vi "SFCT Motor Control.vi"(9 "Start":bool, 10 "VISA resource":refnum<visa-resource-name>, 11 "To Position":u16(ring) items=["Staging", "Press", "Cooling", "Auto Home", "Home"]) -> (0 "Y position":dbl, 1 "X Position":dbl)   [LabVIEW 2020]
uses:
  <vilib>/LabVIEW Interface for Arduino/LabVIEW Interface for Arduino.lvlib
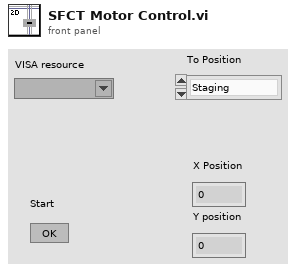
[diagram p1: front panel]
types:
  T1 = typedef "LabVIEW Interface for Arduino.lvlib/Arduino Resource.ctl" = cluster{"VISA resource":refnum<visa-resource-name>, "Board Type":T2, "Connection Type":enum8{"USB / Serial"}, "Bytes Per Packet (15)":u8}
  T2 = typedef "LabVIEW Interface for Arduino.lvlib/Board Type.ctl" = enum16{"Uno", "Dimuelanove w/Atmega 328", "Mega 2560"}
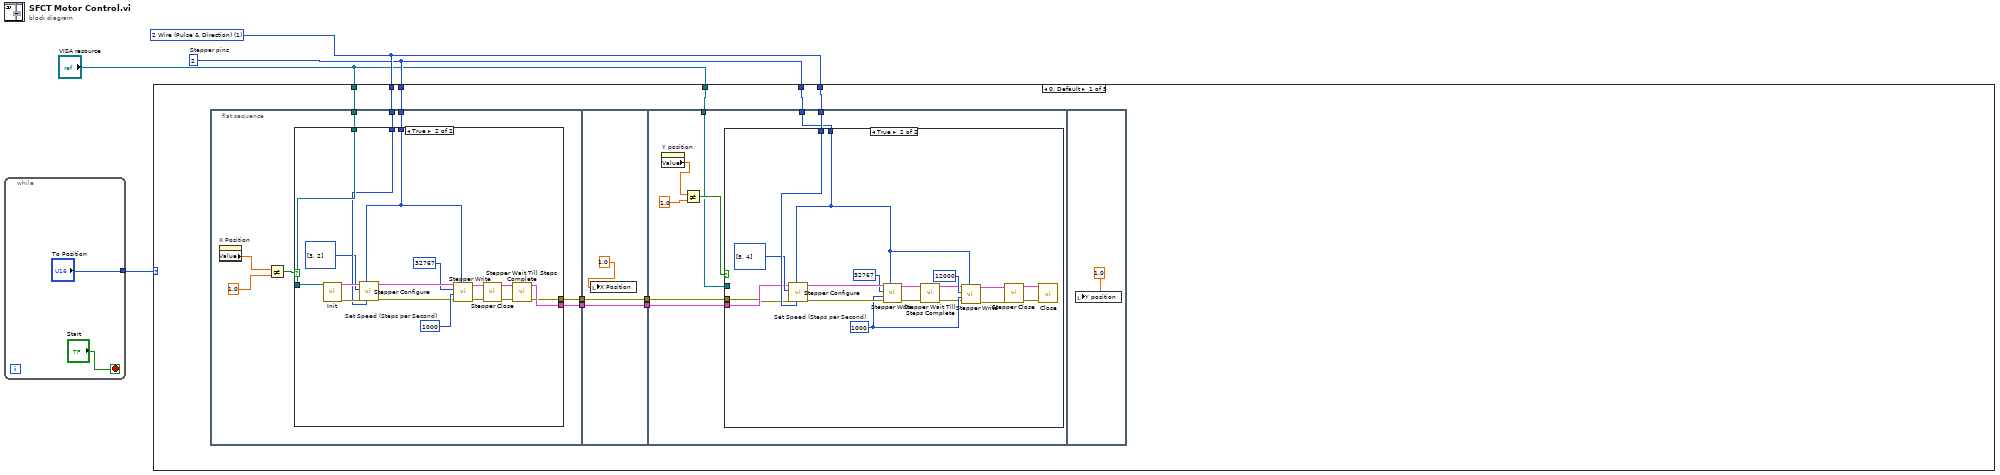
[diagram p0: block diagram]
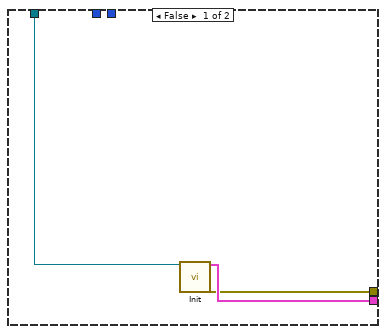
[diagram p2: hidden frame]
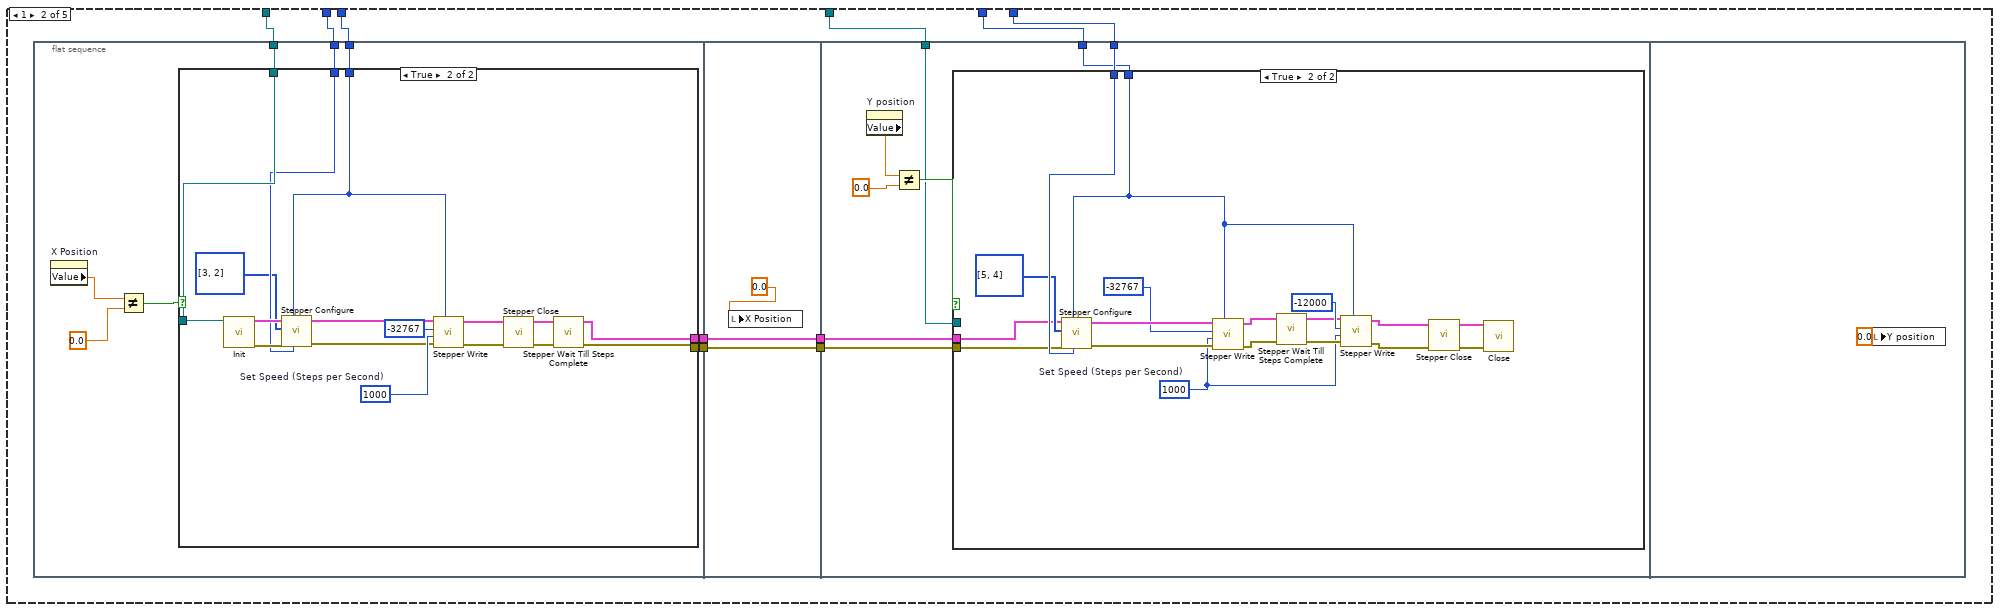
[diagram p4: hidden frame]
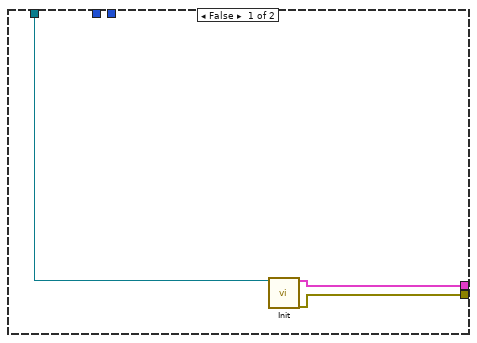
[diagram p5: hidden frame]
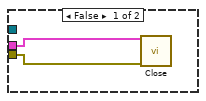
[diagram p6: hidden frame]
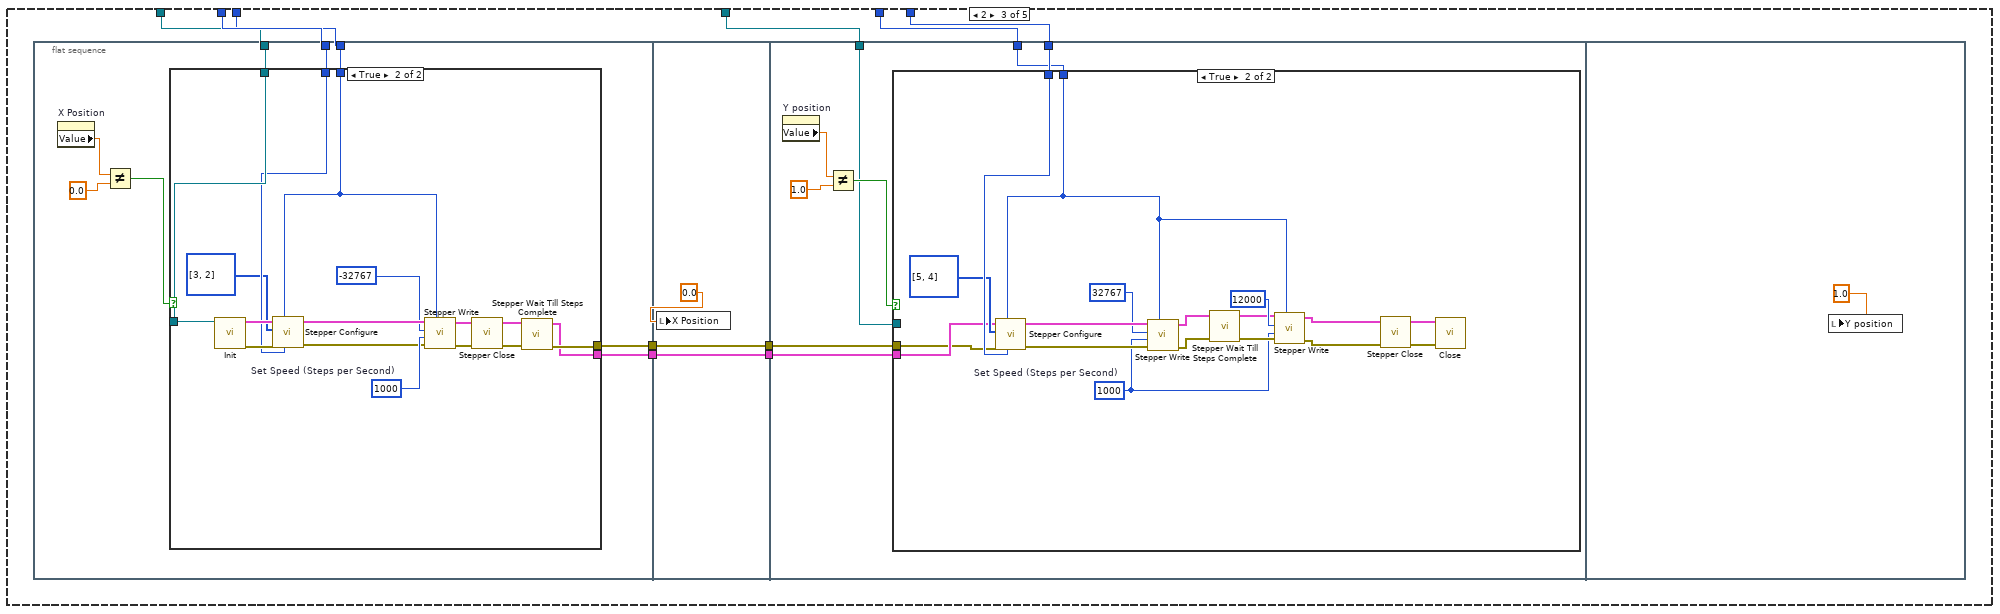
[diagram p7: hidden frame]
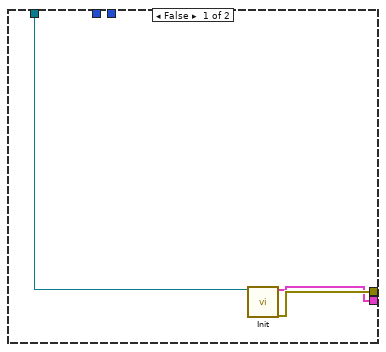
[diagram p8: hidden frame]
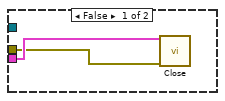
[diagram p9: hidden frame]
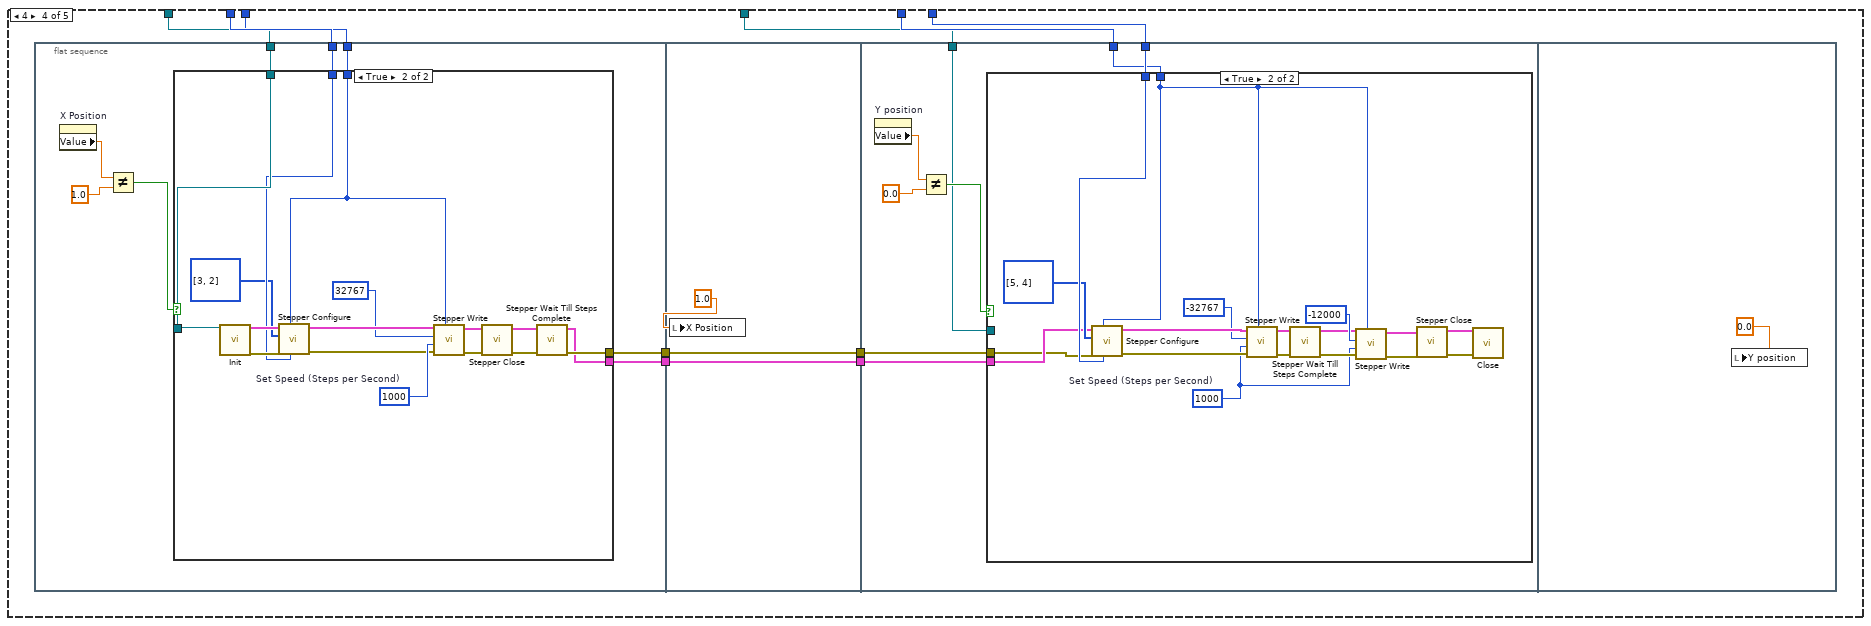
[diagram p10: hidden frame]
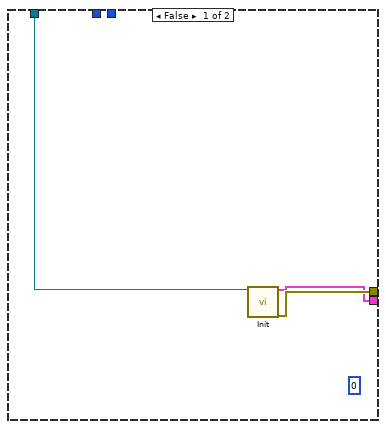
[diagram p11: hidden frame]
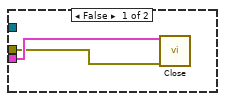
[diagram p12: hidden frame]
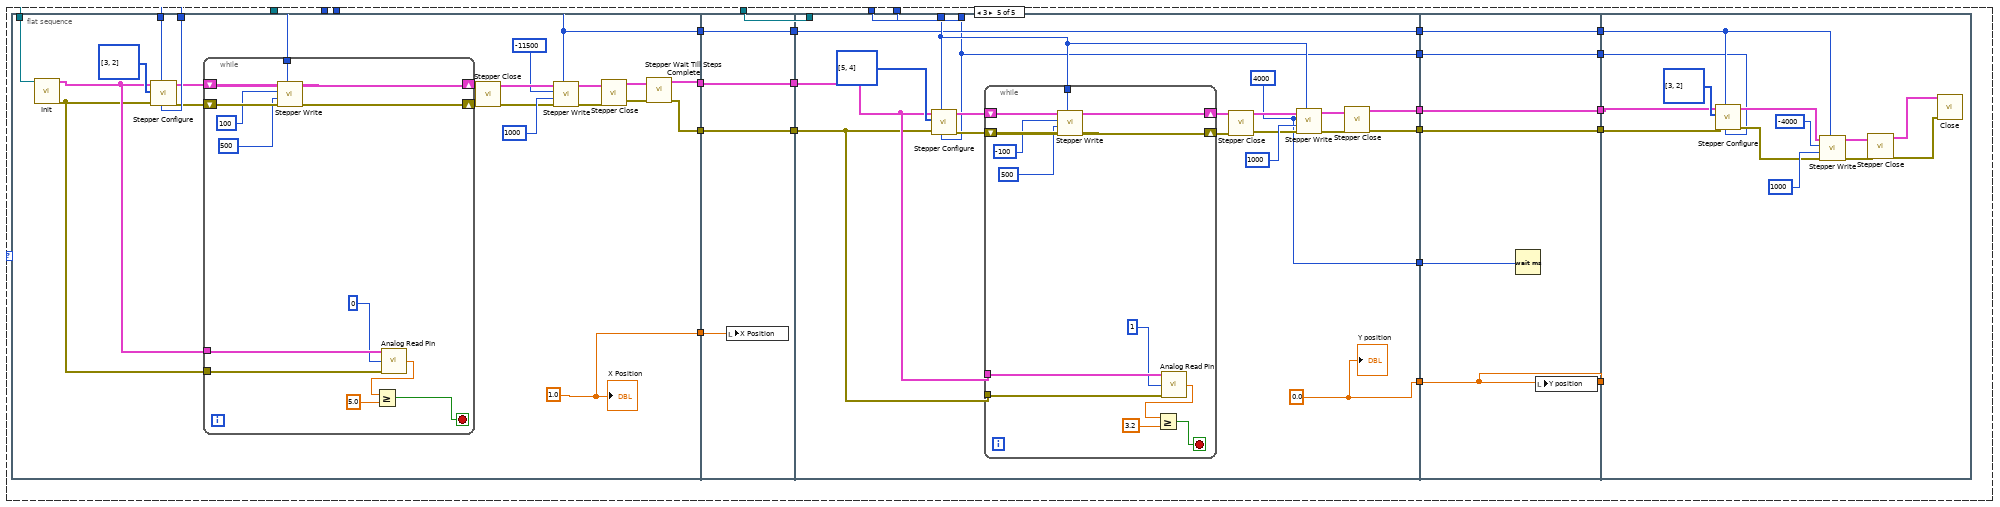
[diagram p13: hidden frame]
diagram:
  w2 = 2  # Stepper pins
  w3 = u8 1 items=["2 Wire (Pulse & Direction)"=1, "2 Wire"=2, "4 Wire"=4, "EasyDriver"=6, "AF Motor Shield (Stepper 1 & 2 Only)"=5] ("Control Method")
  n1 = while {
    tunnel: ["To Position"] -> w4
    stop <- "Start" stop-if-true
  }
  n2 = case shown="0, Default" w4 {
    tunnel: "VISA resource" -> [w11 w78 w147 w216 w301]
    tunnel: w3 -> [w13 w80 w149 w218 w300]
    tunnel: w2 -> [w12 w79 w148 w217 w299]
    tunnel: w3 -> [w16 w83 w152 w221 _]
    tunnel: w2 -> [w15 w82 w151 w220 _]
    tunnel: "VISA resource" -> [w14 w81 w150 w219 _]
    frame 0, Default {
      n3 = flat-sequence {
        tunnel: w16 -> [w23]
        tunnel: w15 -> [w22]
        tunnel: w14 -> [w19]
        tunnel: [w21] -> w9
        tunnel: [w20] -> w7
        tunnel: [w46] -> w10
        tunnel: w9 -> [w46]
        tunnel: [w45] -> w8
        tunnel: w7 -> [w45]
        tunnel: w13 -> [w53]
        tunnel: w12 -> [w52]
        tunnel: w11 -> [w51]
        tunnel: w10 -> [w50]
        tunnel: w8 -> [w49]
        frame #0 {
          n4 = property on="X Position" class="DigNum (strict)"() -> ("Value"=w17:dbl)  [unwired: 2 in, 2 out]
          n5 = Not Equal?(x=w17, y=1.0) -> (x != y?=w24:bool)
          n6 = case shown="True" w24 {
            tunnel: w23 -> [_ w40]
            tunnel: w22 -> [_ w36]
            tunnel: w19 -> [_ w33]
            tunnel: [w27 w31] -> w21
            tunnel: [w26 w30] -> w20
            tunnel: w19 -> [w25 _]
            frame False {
              n7 = call <vilib>:"Init.vi"("VISA resource"=w25) -> ("Arduino Resource"=w27:T1, "error out"=w26:errorcluster)  [unwired: 17 in]
            }
            frame True {
              w41 = i16 1000  # Set Speed (Steps per Second)
              n8 = call <vilib>:"Init.vi"("VISA resource"=w33) -> ("Arduino Resource"=w43:T1, "error out"=w42:errorcluster)  [unwired: 17 in]
              n9 = call <vilib>:"Stepper Configure.vi"("Control Method"=w40, "Stepper #"=w36, "error in"=w42, "Stepper Pins"=u8[] [3, 2], "Arduino Resource"=w43) -> ("error out"=w37:errorcluster, "Arduino Resource Out"=w38:T1)  [unwired: 5 in]
              n10 = call <vilib>:"Stepper Write.vi"("Stepper #"=w36, "error in"=w37, "Set Speed (Steps per Second)"=w41, "# of Steps to Move"=i16 32767, "Arduino Resource"=w38) -> ("error out"=w35:errorcluster, "Arduino Resource Out"=w34:T1)  [unwired: 5 in]
              n11 = call <vilib>:"Stepper Close.vi"("error in"=w35, "Arduino Resource"=w34) -> ("error out"=w29:errorcluster, "Arduino Resource Out"=w28:T1)  [unwired: 8 in]
              n12 = call <vilib>:"Stepper Wait Till Steps Complete.vi"("error in"=w29, "Arduino Resource In"=w28) -> ("error out"=w30:errorcluster, "Arduino Resource Out"=w31:T1)  [unwired: 8 in]
            }
          }
        }
        frame #1 {
          n13 = local write "X Position"(1.0 ("X Position")) -> ()
        }
        frame #2 {
          n14 = property on="Y position" class="DigNum (strict)"() -> ("Value"=w47:dbl)  [unwired: 2 in, 2 out]
          n15 = Not Equal?(x=w47, y=1.0) -> (x != y?=w54:bool)
          n16 = case shown="True" w54 {
            tunnel: w53 -> [_ w72]
            tunnel: w52 -> [_ w61]
            tunnel: w51 -> [_ _]
            tunnel: w50 -> [_ w66]
            tunnel: w49 -> [_ w65]
            frame False {
            }
            frame True {
              w60 = i16 1000  # Set Speed (Steps per Second)
              n17 = call <vilib>:"Stepper Configure.vi"("Control Method"=w72, "Stepper #"=w61, "error in"=w65, "Stepper Pins"=u8[] [5, 4], "Arduino Resource"=w66) -> ("error out"=w69:errorcluster, "Arduino Resource Out"=w70:T1)  [unwired: 5 in]
              n18 = call <vilib>:"Stepper Write.vi"("Stepper #"=w61, "error in"=w69, "Set Speed (Steps per Second)"=w60, "# of Steps to Move"=i16 32767, "Arduino Resource"=w70) -> ("error out"=w58:errorcluster, "Arduino Resource Out"=w57:T1)  [unwired: 5 in]
              n19 = call <vilib>:"Stepper Wait Till Steps Complete.vi"("error in"=w58, "Arduino Resource In"=w57) -> ("error out"=w55:errorcluster, "Arduino Resource Out"=w56:T1)  [unwired: 8 in]
              n20 = call <vilib>:"Stepper Write.vi"("Stepper #"=w61, "error in"=w55, "Set Speed (Steps per Second)"=w60, "# of Steps to Move"=i16 12000, "Arduino Resource"=w56) -> ("error out"=w63:errorcluster, "Arduino Resource Out"=w62:T1)  [unwired: 5 in]
              n21 = call <vilib>:"Stepper Close.vi"("error in"=w63, "Arduino Resource"=w62) -> ("error out"=w67:errorcluster, "Arduino Resource Out"=w68:T1)  [unwired: 8 in]
              n22 = call <vilib>:"Close.vi"("Arduino Resource"=w68, "error in"=w67) -> ()  [unwired: 13 in, 1 out]
            }
          }
        }
        frame #3 {
          n23 = local write "Y position"(1.0 ("Y position")) -> ()
        }
      }
    }
    frame 1 {
      n24 = flat-sequence {
        tunnel: w83 -> [w90]
        tunnel: w82 -> [w89]
        tunnel: w81 -> [w86]
        tunnel: [w88] -> w76
        tunnel: [w87] -> w74
        tunnel: [w113] -> w77
        tunnel: w76 -> [w113]
        tunnel: [w112] -> w75
        tunnel: w74 -> [w112]
        tunnel: w80 -> [w120]
        tunnel: w79 -> [w119]
        tunnel: w78 -> [w118]
        tunnel: w77 -> [w117]
        tunnel: w75 -> [w116]
        frame #0 {
          n25 = property on="X Position" class="DigNum (strict)"() -> ("Value"=w84:dbl)  [unwired: 2 in, 2 out]
          n26 = Not Equal?(x=w84, y=0.0) -> (x != y?=w91:bool)
          n27 = case shown="True" w91 {
            tunnel: w90 -> [_ w107]
            tunnel: w89 -> [_ w103]
            tunnel: w86 -> [_ w100]
            tunnel: [w92 w95] -> w88
            tunnel: [w93 w96] -> w87
            tunnel: w86 -> [w94 _]
            frame False {
              n28 = call <vilib>:"Init.vi"("VISA resource"=w94) -> ("Arduino Resource"=w93:T1, "error out"=w92:errorcluster)  [unwired: 17 in]
            }
            frame True {
              w108 = i16 1000  # Set Speed (Steps per Second)
              n29 = call <vilib>:"Init.vi"("VISA resource"=w100) -> ("Arduino Resource"=w110:T1, "error out"=w109:errorcluster)  [unwired: 17 in]
              n30 = call <vilib>:"Stepper Configure.vi"("Control Method"=w107, "Stepper #"=w103, "error in"=w109, "Stepper Pins"=u8[] [3, 2], "Arduino Resource"=w110) -> ("error out"=w104:errorcluster, "Arduino Resource Out"=w105:T1)  [unwired: 5 in]
              n31 = call <vilib>:"Stepper Write.vi"("Stepper #"=w103, "error in"=w104, "Set Speed (Steps per Second)"=w108, "# of Steps to Move"=i16 -32767, "Arduino Resource"=w105) -> ("error out"=w102:errorcluster, "Arduino Resource Out"=w101:T1)  [unwired: 5 in]
              n32 = call <vilib>:"Stepper Close.vi"("error in"=w102, "Arduino Resource"=w101) -> ("error out"=w97:errorcluster, "Arduino Resource Out"=w98:T1)  [unwired: 8 in]
              n33 = call <vilib>:"Stepper Wait Till Steps Complete.vi"("error in"=w97, "Arduino Resource In"=w98) -> ("error out"=w95:errorcluster, "Arduino Resource Out"=w96:T1)  [unwired: 8 in]
            }
          }
        }
        frame #1 {
          n34 = local write "X Position"(0.0 ("X Position")) -> ()
        }
        frame #2 {
          n35 = property on="Y position" class="DigNum (strict)"() -> ("Value"=w114:dbl)  [unwired: 2 in, 2 out]
          n36 = Not Equal?(x=w114, y=0.0) -> (x != y?=w121:bool)
          n37 = case shown="True" w121 {
            tunnel: w120 -> [_ w141]
            tunnel: w119 -> [_ w125]
            tunnel: w118 -> [_ _]
            tunnel: w117 -> [w122 w135]
            tunnel: w116 -> [w123 w134]
            frame False {
              n38 = call <vilib>:"Close.vi"("Arduino Resource"=w123, "error in"=w122) -> ()  [unwired: 13 in, 1 out]
            }
            frame True {
              w124 = i16 1000  # Set Speed (Steps per Second)
              n39 = call <vilib>:"Stepper Configure.vi"("Control Method"=w141, "Stepper #"=w125, "error in"=w135, "Stepper Pins"=u8[] [5, 4], "Arduino Resource"=w134) -> ("error out"=w138:errorcluster, "Arduino Resource Out"=w139:T1)  [unwired: 5 in]
              n40 = call <vilib>:"Stepper Write.vi"("Stepper #"=w125, "error in"=w138, "Set Speed (Steps per Second)"=w124, "# of Steps to Move"=i16 -32767, "Arduino Resource"=w139) -> ("error out"=w128:errorcluster, "Arduino Resource Out"=w129:T1)  [unwired: 5 in]
              n41 = call <vilib>:"Stepper Wait Till Steps Complete.vi"("error in"=w128, "Arduino Resource In"=w129) -> ("error out"=w130:errorcluster, "Arduino Resource Out"=w131:T1)  [unwired: 8 in]
              n42 = call <vilib>:"Stepper Write.vi"("Stepper #"=w125, "error in"=w130, "Set Speed (Steps per Second)"=w124, "# of Steps to Move"=i16 -12000, "Arduino Resource"=w131) -> ("error out"=w127:errorcluster, "Arduino Resource Out"=w126:T1)  [unwired: 5 in]
              n43 = call <vilib>:"Stepper Close.vi"("error in"=w127, "Arduino Resource"=w126) -> ("error out"=w136:errorcluster, "Arduino Resource Out"=w137:T1)  [unwired: 8 in]
              n44 = call <vilib>:"Close.vi"("Arduino Resource"=w137, "error in"=w136) -> ()  [unwired: 13 in, 1 out]
            }
          }
        }
        frame #3 {
          n45 = local write "Y position"(0.0 ("Y position")) -> ()
        }
      }
    }
    frame 2 {
      n46 = flat-sequence {
        tunnel: w152 -> [w159]
        tunnel: w151 -> [w158]
        tunnel: w150 -> [w155]
        tunnel: [w157] -> w145
        tunnel: [w156] -> w144
        tunnel: [w182] -> w146
        tunnel: w145 -> [w182]
        tunnel: w144 -> [w181]
        tunnel: [w181] -> w143
        tunnel: w149 -> [w189]
        tunnel: w148 -> [w188]
        tunnel: w147 -> [w187]
        tunnel: w146 -> [w186]
        tunnel: w143 -> [w185]
        frame #0 {
          n47 = property on="X Position" class="DigNum (strict)"() -> ("Value"=w153:dbl)  [unwired: 2 in, 2 out]
          n48 = Not Equal?(x=w153, y=0.0) -> (x != y?=w160:bool)
          n49 = case shown="True" w160 {
            tunnel: w159 -> [_ w176]
            tunnel: w158 -> [_ w172]
            tunnel: w155 -> [_ w169]
            tunnel: [w162 w164] -> w157
            tunnel: [w163 w165] -> w156
            tunnel: w155 -> [w161 _]
            frame False {
              n50 = call <vilib>:"Init.vi"("VISA resource"=w161) -> ("Arduino Resource"=w162:T1, "error out"=w163:errorcluster)  [unwired: 17 in]
            }
            frame True {
              w177 = i16 1000  # Set Speed (Steps per Second)
              n51 = call <vilib>:"Init.vi"("VISA resource"=w169) -> ("Arduino Resource"=w179:T1, "error out"=w178:errorcluster)  [unwired: 17 in]
              n52 = call <vilib>:"Stepper Configure.vi"("Control Method"=w176, "Stepper #"=w172, "error in"=w178, "Stepper Pins"=u8[] [3, 2], "Arduino Resource"=w179) -> ("error out"=w173:errorcluster, "Arduino Resource Out"=w174:T1)  [unwired: 5 in]
              n53 = call <vilib>:"Stepper Write.vi"("Stepper #"=w172, "error in"=w173, "Set Speed (Steps per Second)"=w177, "# of Steps to Move"=i16 -32767, "Arduino Resource"=w174) -> ("error out"=w171:errorcluster, "Arduino Resource Out"=w170:T1)  [unwired: 5 in]
              n54 = call <vilib>:"Stepper Close.vi"("error in"=w171, "Arduino Resource"=w170) -> ("error out"=w166:errorcluster, "Arduino Resource Out"=w167:T1)  [unwired: 8 in]
              n55 = call <vilib>:"Stepper Wait Till Steps Complete.vi"("error in"=w166, "Arduino Resource In"=w167) -> ("error out"=w165:errorcluster, "Arduino Resource Out"=w164:T1)  [unwired: 8 in]
            }
          }
        }
        frame #1 {
          n56 = local write "X Position"(0.0 ("X Position")) -> ()
        }
        frame #2 {
          n57 = property on="Y position" class="DigNum (strict)"() -> ("Value"=w183:dbl)  [unwired: 2 in, 2 out]
          n58 = Not Equal?(x=w183, y=1.0) -> (x != y?=w190:bool)
          n59 = case shown="True" w190 {
            tunnel: w189 -> [_ w210]
            tunnel: w188 -> [_ w194]
            tunnel: w187 -> [_ _]
            tunnel: w186 -> [w192 w204]
            tunnel: w185 -> [w191 w203]
            frame False {
              n60 = call <vilib>:"Close.vi"("Arduino Resource"=w192, "error in"=w191) -> ()  [unwired: 13 in, 1 out]
            }
            frame True {
              w193 = i16 1000  # Set Speed (Steps per Second)
              n61 = call <vilib>:"Stepper Configure.vi"("Control Method"=w210, "Stepper #"=w194, "error in"=w203, "Stepper Pins"=u8[] [5, 4], "Arduino Resource"=w204) -> ("error out"=w207:errorcluster, "Arduino Resource Out"=w208:T1)  [unwired: 5 in]
              n62 = call <vilib>:"Stepper Write.vi"("Stepper #"=w194, "error in"=w207, "Set Speed (Steps per Second)"=w193, "# of Steps to Move"=i16 32767, "Arduino Resource"=w208) -> ("error out"=w197:errorcluster, "Arduino Resource Out"=w198:T1)  [unwired: 5 in]
              n63 = call <vilib>:"Stepper Wait Till Steps Complete.vi"("error in"=w197, "Arduino Resource In"=w198) -> ("error out"=w199:errorcluster, "Arduino Resource Out"=w200:T1)  [unwired: 8 in]
              n64 = call <vilib>:"Stepper Write.vi"("Stepper #"=w194, "error in"=w199, "Set Speed (Steps per Second)"=w193, "# of Steps to Move"=i16 12000, "Arduino Resource"=w200) -> ("error out"=w195:errorcluster, "Arduino Resource Out"=w196:T1)  [unwired: 5 in]
              n65 = call <vilib>:"Stepper Close.vi"("error in"=w195, "Arduino Resource"=w196) -> ("error out"=w205:errorcluster, "Arduino Resource Out"=w206:T1)  [unwired: 8 in]
              n66 = call <vilib>:"Close.vi"("Arduino Resource"=w206, "error in"=w205) -> ()  [unwired: 13 in, 1 out]
            }
          }
        }
        frame #3 {
          n67 = local write "Y position"(1.0 ("Y position")) -> ()
        }
      }
    }
    frame 4 {
      n68 = flat-sequence {
        tunnel: w221 -> [w228]
        tunnel: w220 -> [w227]
        tunnel: w219 -> [w224]
        tunnel: [w226] -> w214
        tunnel: [w225] -> w213
        tunnel: [w251] -> w215
        tunnel: w214 -> [w251]
        tunnel: w213 -> [w250]
        tunnel: [w250] -> w212
        tunnel: w218 -> [w258]
        tunnel: w217 -> [w257]
        tunnel: w216 -> [w256]
        tunnel: w215 -> [w255]
        tunnel: w212 -> [w254]
        frame #0 {
          n69 = property on="X Position" class="DigNum (strict)"() -> ("Value"=w222:dbl)  [unwired: 2 in, 2 out]
          n70 = Not Equal?(x=w222, y=1.0) -> (x != y?=w229:bool)
          n71 = case shown="True" w229 {
            tunnel: w228 -> [_ w245]
            tunnel: w227 -> [_ w241]
            tunnel: w224 -> [_ w238]
            tunnel: [w231 w233] -> w226
            tunnel: [w232 w234] -> w225
            tunnel: w224 -> [w230 _]
            frame False {
              (unwired) i16 0 ("# of Steps to Move")
              n72 = call <vilib>:"Init.vi"("VISA resource"=w230) -> ("Arduino Resource"=w231:T1, "error out"=w232:errorcluster)  [unwired: 17 in]
            }
            frame True {
              w246 = i16 1000  # Set Speed (Steps per Second)
              n73 = call <vilib>:"Init.vi"("VISA resource"=w238) -> ("Arduino Resource"=w248:T1, "error out"=w247:errorcluster)  [unwired: 17 in]
              n74 = call <vilib>:"Stepper Configure.vi"("Control Method"=w245, "Stepper #"=w241, "error in"=w247, "Stepper Pins"=u8[] [3, 2], "Arduino Resource"=w248) -> ("error out"=w242:errorcluster, "Arduino Resource Out"=w243:T1)  [unwired: 5 in]
              n75 = call <vilib>:"Stepper Write.vi"("Stepper #"=w241, "error in"=w242, "Set Speed (Steps per Second)"=w246, "# of Steps to Move"=i16 32767, "Arduino Resource"=w243) -> ("error out"=w240:errorcluster, "Arduino Resource Out"=w239:T1)  [unwired: 5 in]
              n76 = call <vilib>:"Stepper Close.vi"("error in"=w240, "Arduino Resource"=w239) -> ("error out"=w235:errorcluster, "Arduino Resource Out"=w236:T1)  [unwired: 8 in]
              n77 = call <vilib>:"Stepper Wait Till Steps Complete.vi"("error in"=w235, "Arduino Resource In"=w236) -> ("error out"=w234:errorcluster, "Arduino Resource Out"=w233:T1)  [unwired: 8 in]
            }
          }
        }
        frame #1 {
          n78 = local write "X Position"(1.0 ("X Position")) -> ()
        }
        frame #2 {
          n79 = property on="Y position" class="DigNum (strict)"() -> ("Value"=w252:dbl)  [unwired: 2 in, 2 out]
          n80 = Not Equal?(x=w252, y=0.0) -> (x != y?=w259:bool)
          n81 = case shown="True" w259 {
            tunnel: w258 -> [_ w279]
            tunnel: w257 -> [_ w263]
            tunnel: w256 -> [_ _]
            tunnel: w255 -> [w261 w274]
            tunnel: w254 -> [w260 w273]
            frame False {
              n82 = call <vilib>:"Close.vi"("Arduino Resource"=w261, "error in"=w260) -> ()  [unwired: 13 in, 1 out]
            }
            frame True {
              w262 = i16 1000  # Set Speed (Steps per Second)
              n83 = call <vilib>:"Stepper Configure.vi"("Control Method"=w279, "Stepper #"=w263, "error in"=w273, "Stepper Pins"=u8[] [5, 4], "Arduino Resource"=w274) -> ("error out"=w277:errorcluster, "Arduino Resource Out"=w272:T1)  [unwired: 5 in]
              n84 = call <vilib>:"Stepper Write.vi"("Stepper #"=w263, "error in"=w277, "Set Speed (Steps per Second)"=w262, "# of Steps to Move"=i16 -32767, "Arduino Resource"=w272) -> ("error out"=w266:errorcluster, "Arduino Resource Out"=w267:T1)  [unwired: 5 in]
              n85 = call <vilib>:"Stepper Wait Till Steps Complete.vi"("error in"=w266, "Arduino Resource In"=w267) -> ("error out"=w268:errorcluster, "Arduino Resource Out"=w269:T1)  [unwired: 8 in]
              n86 = call <vilib>:"Stepper Write.vi"("Stepper #"=w263, "error in"=w268, "Set Speed (Steps per Second)"=w262, "# of Steps to Move"=i16 -12000, "Arduino Resource"=w269) -> ("error out"=w264:errorcluster, "Arduino Resource Out"=w265:T1)  [unwired: 5 in]
              n87 = call <vilib>:"Stepper Close.vi"("error in"=w264, "Arduino Resource"=w265) -> ("error out"=w275:errorcluster, "Arduino Resource Out"=w276:T1)  [unwired: 8 in]
              n88 = call <vilib>:"Close.vi"("Arduino Resource"=w276, "error in"=w275) -> ()  [unwired: 13 in, 1 out]
            }
          }
        }
        frame #3 {
          n89 = local write "Y position"(0.0 ("Y position")) -> ()
        }
      }
    }
    frame 3 {
      n90 = flat-sequence {
        tunnel: w301 -> [w322]
        tunnel: w300 -> [w321]
        tunnel: w299 -> [w306]
        tunnel: [w308] -> w298
        tunnel: [w305] -> w296
        tunnel: [w304] -> w294
        tunnel: [w306] -> w287
        tunnel: w298 -> [w339]
        tunnel: [w338] -> w297
        tunnel: w296 -> [w338]
        tunnel: [w337] -> w295
        tunnel: w294 -> [w337]
        tunnel: [w336] -> w288
        tunnel: w287 -> [w336]
        tunnel: w301 -> [_]
        tunnel: w300 -> [w340]
        tunnel: w299 -> [w348]
        tunnel: w297 -> [w347]
        tunnel: w295 -> [w346]
        tunnel: [w345] -> w293
        tunnel: [w344] -> w291
        tunnel: [w343] -> w290
        tunnel: [w342] -> w289
        tunnel: w288 -> [w342]
        tunnel: [w341] -> w283
        tunnel: [w340] -> w282
        tunnel: w293 -> [w377]
        tunnel: [w377] -> w292
        tunnel: w291 -> [w374]
        tunnel: w290 -> [w375]
        tunnel: w289 -> [w376]
        tunnel: [w376] -> w286
        tunnel: [w375] -> w285
        tunnel: [w374] -> w284
        tunnel: w283 -> [w373]
        tunnel: w282 -> [w372]
        tunnel: [w372] -> w281
        tunnel: w292 -> [_]
        tunnel: w286 -> [w379]
        tunnel: w285 -> [w383]
        tunnel: w284 -> [w380]
        tunnel: w281 -> [w378]
        frame #0 {
          w308 = 1.0
          n91 = call <vilib>:"Init.vi"("VISA resource"=w322) -> ("Arduino Resource"=w310:T1, "error out"=w309:errorcluster)  [unwired: 17 in]
          n92 = call <vilib>:"Stepper Configure.vi"("Control Method"=w321, "Stepper #"=w306, "error in"=w309, "Stepper Pins"=u8[] [3, 2], "Arduino Resource"=w310) -> ("error out"=w311:errorcluster, "Arduino Resource Out"=w312:T1)  [unwired: 5 in]
          n93 = while {
            tunnel: w310 -> [w335]
            tunnel: w309 -> [w334]
            shift-right: [w331] -> w315
            shift-left: w312 -> [w333]
            shift-right: [w330] -> w316
            shift-left: w311 -> [w332]
            tunnel: w306 -> [w329]
            stop <- w325 stop-if-true
            n94 = call <vilib>:"Stepper Write.vi"("Stepper #"=w329, "error in"=w332, "Set Speed (Steps per Second)"=i16 500, "# of Steps to Move"=i16 100, "Arduino Resource"=w333) -> ("error out"=w330:errorcluster, "Arduino Resource Out"=w331:T1)  [unwired: 5 in]
            n95 = call <vilib>:"Analog Read Pin.vi"("Arduino Resource"=w335, "Analog Input Pin (0)"=u8 0, "error in"=w334) -> ("Voltage"=w324:dbl)  [unwired: 10 in, 2 out]
            n96 = Greater Or Equal?(x=w324, y=5.0) -> (x >= y?=w325:bool)
          }
          n97 = call <vilib>:"Stepper Close.vi"("error in"=w316, "Arduino Resource"=w315) -> ("error out"=w317:errorcluster, "Arduino Resource Out"=w318:T1)  [unwired: 8 in]
          n98 = call <vilib>:"Stepper Write.vi"("Stepper #"=w306, "error in"=w317, "Set Speed (Steps per Second)"=i16 1000, "# of Steps to Move"=i16 -11500, "Arduino Resource"=w318) -> ("error out"=w314:errorcluster, "Arduino Resource Out"=w313:T1)  [unwired: 5 in]
          n99 = call <vilib>:"Stepper Close.vi"("error in"=w314, "Arduino Resource"=w313) -> ("error out"=w303:errorcluster, "Arduino Resource Out"=w302:T1)  [unwired: 8 in]
          n100 = call <vilib>:"Stepper Wait Till Steps Complete.vi"("error in"=w303, "Arduino Resource In"=w302) -> ("error out"=w304:errorcluster, "Arduino Resource Out"=w305:T1)  [unwired: 8 in]
          "X Position" <- w308
        }
        frame #1 {
          n101 = local write "X Position"(w339) -> ()
        }
        frame #2 {
          w345 = 0.0
          w341 = i16 4000 ("# of Steps to Move")
          n102 = call <vilib>:"Stepper Configure.vi"("Control Method"=w340, "Stepper #"=w348, "error in"=w346, "Stepper Pins"=u8[] [5, 4], "Arduino Resource"=w347) -> ("error out"=w349:errorcluster, "Arduino Resource Out"=w350:T1)  [unwired: 5 in]
          n103 = while {
            tunnel: w347 -> [w371]
            tunnel: w346 -> [w370]
            shift-right: [w367] -> w353
            shift-left: w350 -> [w369]
            shift-right: [w366] -> w354
            shift-left: w349 -> [w368]
            tunnel: w348 -> [w365]
            stop <- w360 stop-if-true
            n104 = call <vilib>:"Stepper Write.vi"("Stepper #"=w365, "error in"=w368, "Set Speed (Steps per Second)"=i16 500, "# of Steps to Move"=i16 -100, "Arduino Resource"=w369) -> ("error out"=w366:errorcluster, "Arduino Resource Out"=w367:T1)  [unwired: 5 in]
            n105 = call <vilib>:"Analog Read Pin.vi"("Arduino Resource"=w371, "Analog Input Pin (0)"=u8 1, "error in"=w370) -> ("Voltage"=w359:dbl)  [unwired: 10 in, 2 out]
            n106 = Greater Or Equal?(x=w359, y=3.2) -> (x >= y?=w360:bool)
          }
          n107 = call <vilib>:"Stepper Close.vi"("error in"=w354, "Arduino Resource"=w353) -> ("error out"=w355:errorcluster, "Arduino Resource Out"=w356:T1)  [unwired: 8 in]
          n108 = call <vilib>:"Stepper Write.vi"("Stepper #"=w348, "error in"=w355, "Set Speed (Steps per Second)"=i16 1000, "# of Steps to Move"=w341, "Arduino Resource"=w356) -> ("error out"=w352:errorcluster, "Arduino Resource Out"=w351:T1)  [unwired: 5 in]
          n109 = call <vilib>:"Stepper Close.vi"("error in"=w352, "Arduino Resource"=w351) -> ("error out"=w343:errorcluster, "Arduino Resource Out"=w344:T1)  [unwired: 8 in]
          "Y position" <- w345
        }
        frame #3 {
          n110 = Wait (ms)(milliseconds to wait=w373) -> ()  [unwired: 1 out]
          n111 = local write "Y position"(w377) -> ()
        }
        frame #4 {
          n112 = call <vilib>:"Stepper Configure.vi"("Control Method"=w378, "Stepper #"=w379, "error in"=w383, "Stepper Pins"=u8[] [3, 2], "Arduino Resource"=w380) -> ("error out"=w382:errorcluster, "Arduino Resource Out"=w381:T1)  [unwired: 5 in]
          n113 = call <vilib>:"Stepper Write.vi"("Stepper #"=w379, "error in"=w382, "Set Speed (Steps per Second)"=i16 1000, "# of Steps to Move"=i16 -4000, "Arduino Resource"=w381) -> ("error out"=w387:errorcluster, "Arduino Resource Out"=w388:T1)  [unwired: 5 in]
          n114 = call <vilib>:"Stepper Close.vi"("error in"=w387, "Arduino Resource"=w388) -> ("error out"=w390:errorcluster, "Arduino Resource Out"=w389:T1)  [unwired: 8 in]
          n115 = call <vilib>:"Close.vi"("Arduino Resource"=w389, "error in"=w390) -> ()  [unwired: 13 in, 1 out]
        }
      }
    }
  }
